vi "Read Wfm Data.vi"(8 "error in (no error)":errorcluster, 10 "Queue in":refnum<queue>, 11 "Parameters in":T1) -> (0 "error out":errorcluster, 2 "Wfm Data":dbl[][](array[numeric]), 3 "Parameters out":T1)   [LabVIEW 2014, in "Waveform-Processing-Custom-Device Engine.lvlib"]
uses:
  Waveform-Processing-Custom-Device Engine.lvlib
  Types/Async Parameters.ctl
  Types/Async FIFOs.ctl
  <vilib>/NI Veristand/Custom Device Waveform API/Single Waveform Read (DBL)/Single Waveform Read (DBL).lvclass
  <vilib>/NI Veristand/Custom Device Waveform API/NI_VS Custom Device Waveform API.lvlib
  <vilib>/NI Veristand/Custom Device Waveform API/Single Waveform Read (DBL)/NI VeriStand - Read Single Waveform (DBL).vi
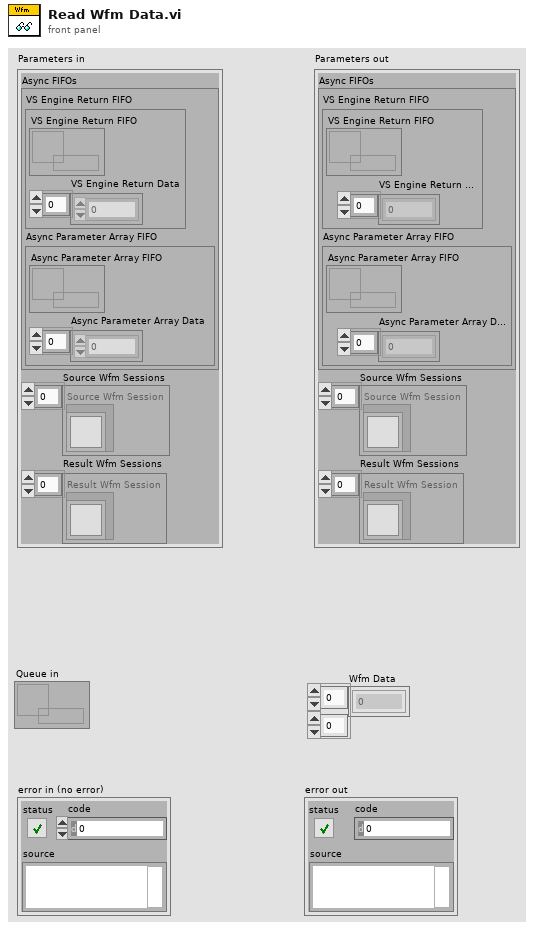
[diagram p1: front panel]
types:
  T1 = typedef "Waveform-Processing-Custom-Device Engine.lvlib/Async Parameters.ctl" = cluster{"Async FIFOs":T2, "Source Wfm Sessions":refnum<class "Single Waveform Read (DBL).lvclass">[], "Result Wfm Sessions":refnum<class "Single Waveform Read (DBL).lvclass">[]}
  T2 = typedef "Waveform-Processing-Custom-Device Engine.lvlib/Async FIFOs.ctl" = cluster{"VS Engine Return FIFO":cluster{"VS Engine Return FIFO":refnum<k33>, "VS Engine Return Data":dbl[]}, "Async Parameter Array FIFO":cluster{"Async Parameter Array FIFO":refnum<k33>, "Async Parameter Array Data":dbl[]}}
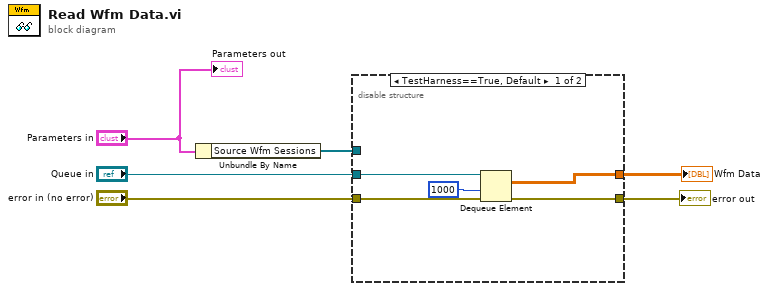
[diagram p0: block diagram]
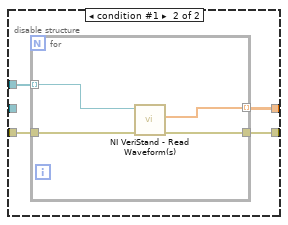
[diagram p2: hidden frame]
diagram:
  n1 = Unbundle By Name("Parameters in") -> ("Source Wfm Sessions"=w6:refnum<class "Single Waveform Read (DBL).lvclass">[])
  n2 = disable-structure shown="TestHarness==True, Default" {
    disable-tunnel: "error in (no error)" -> [w11 w15]
    disable-tunnel: [w10 w14] -> w3
    disable-tunnel: [w9 w13] -> w4
    disable-tunnel: "Queue in" -> [w8 _]
    disable-tunnel: w6 -> [_ w12]
    frame condition #0 (active) {
      n3 = Dequeue Element(queue=w8, timeout in ms (-1)=1000, error in (no error)=w11) -> (element=w9:dbl[][], error out=w10:errorcluster)  [unwired: 2 out]
    }
    frame condition #1 {
      n4 = for {
        tunnel: w15 -> [w19]
        tunnel: [w18] -> w14
        tunnel: [w17] -> w13 mode=indexing
        tunnel: w12 -> [w16] mode=indexing
        n5 = call-poly <vilib>:"NI VeriStand - Read Waveform(s).vi"("error in (no error)"=w19, "Single Waveform Read Session (DBL) in"=w16) -> ("error out"=w18:errorcluster, "Data"=w17:dbl[])  [unwired: 5 in, 3 out]
      }
    }
  }
  "Wfm Data" <- w4
  "error out" <- w3
  "Parameters out" <- "Parameters in"
